vi "Measurement Unit.vi"(4 "Test Input Impedance(T:50 ohm)":bool=TRUE, 6 "Test Attenuation (F:0 dB)":bool, 7 "Power Splitter (F:Dual)":bool, 8 "error in (no error)":errorcluster, 9 "Ref Input Impedance (T:50 ohm)":bool=TRUE, 10 "Ref Attenuation (F:0 dB)":bool, 11 "VISA resource name":refnum<visa-resource-name>) -> (0 "error out":errorcluster, 3 "VISA resource name out":refnum<visa-resource-name>)   [LabVIEW 2017, in "Agilent 4194.lvlib"]
doc: "This function sets the parameters of measurement unit."
uses:
  Agilent 4194.lvlib
panel:
  # "Single\nDual"
  # "20 dB\n0 dB"
  # "50 ohm\n1 Mohm"
  # "20 dB\n0 dB"
  # "50 ohm\n1 Mohm"
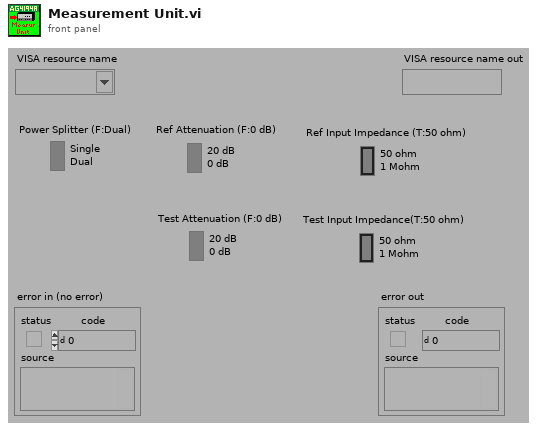
[diagram p1: front panel]
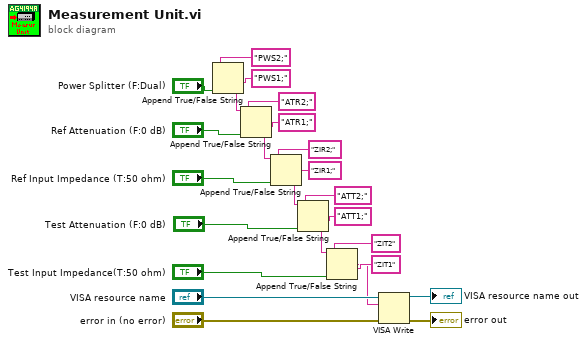
[diagram p0: block diagram]
diagram:
  n1 = Append True/False String(1:"Power Splitter (F:Dual)", 2:"PWS1;", 3:"PWS2;") -> (0:w13:string)  [unwired: 1 in]
  n2 = Append True/False String(1:"Ref Attenuation (F:0 dB)", 2:"ATR1;", 3:"ATR2;", 4:w13) -> (0:w12:string)
  n3 = Append True/False String(1:"Ref Input Impedance (T:50 ohm)", 2:"ZIR1;", 3:"ZIR2;", 4:w12) -> (0:w11:string)
  n4 = Append True/False String(1:"Test Attenuation (F:0 dB)", 2:"ATT1;", 3:"ATT2;", 4:w11) -> (0:w10:string)
  n5 = Append True/False String(1:"Test Input Impedance(T:50 ohm)", 2:"ZIT1", 3:"ZIT2", 4:w10) -> (0:w1:string)
  n6 = VISA Write(VISA resource name="VISA resource name", write buffer=w1, error in (no error)="error in (no error)") -> (VISA resource name out=→"VISA resource name out":refnum<visa-resource-name>, error out=→"error out":errorcluster)  [unwired: 1 out]
